vi "LINX - TMP3x.vi"() -> ()   [LabVIEW 2020]
doc: "Read the temperature from a TMP3x sensor."
uses:
  vi.lib/MakerHub/LINX/Public/Utilities/Open Serial.vi
  vi.lib/MakerHub/LINX/Public/Sensors/Temperature/TMP3x/TMP35.vi
  vi.lib/MakerHub/LINX/LMH-LINX.lvlib
  vi.lib/MakerHub/LINX/Private/Device/Device.lvlib
  vi.lib/MakerHub/LINX/Public/Sensors/Temperature/TMP3x/TMP3x.lvlib
panel:
  out "Temp C":dbl(slide) scale=0.0..35.0
  in  "AI Channel":u8
  out "Loop Rate (Hz)":u32
  in  "Stop Button":bool
  in  "Serial Port":refnum<visa-resource-name>
  # "Circuit Schematic"
  # "LINX Device Settings"
  # "Temperature"
  # "Analog Read Example (Serial Interface)\n\nThis example demonstrates how to read analog input values from a LINX device connected to the host computer via Serial / USB.\n\nInstructions\n1. Select the COM Port associated with the LINX Device.\n2. Select the Analog Channel connected to the TMP3x.\n3. Click the Run Arrow."
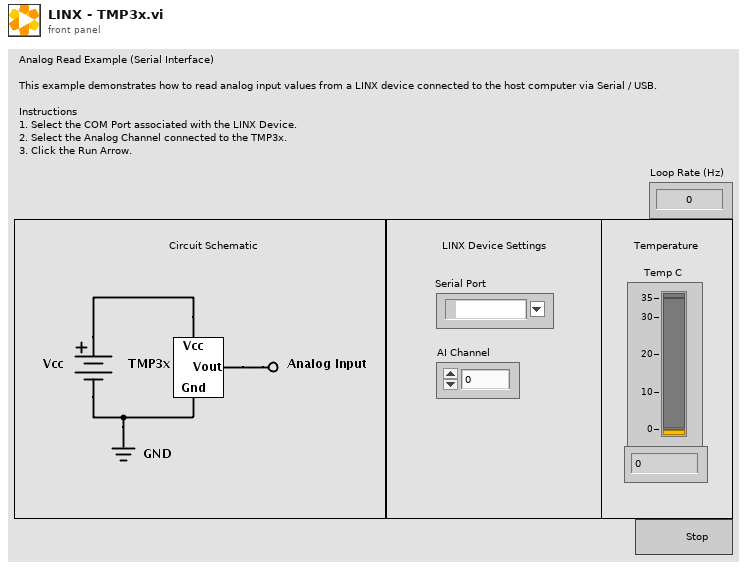
[diagram p1: front panel]
types:
  T1 = typedef "LMH-LINX.lvlib/LINX Ref.ctl" = cluster{"IO":T2, "Interface":T3, "LINX Device Config":T4}
  T2 = typedef "LMH-LINX.lvlib/Platform.ctl" = enum16{"Remote", "Local"}
  T3 = typedef "LMH-LINX.lvlib/Interface.ctl" = enum16{"Serial", "TCP"}
  T4 = typedef "Device.lvlib/LINX Device Config.ctl" = cluster{"Interface":T3, "COM Port":refnum<visa-resource-name>, "TCP Configuration":T5, "Device Family":u8, "Device ID":u8, "Device Name":string, "TCP Ref":refnum<k5>, "Channels":T6}
  T5 = typedef "Device.lvlib/TCP Config.ctl" = cluster{"IP Address":string, "Port":u16}
  T6 = typedef "LMH-LINX.lvlib/Channels.ctl" = cluster{"DI":u8[], "DO":u8[], "AI":u8[], "AO":u8[], "PWM":u8[], "QE":u8[], "UART":u8[], "I2C 2":u8[], "SPI":u8[], "CAN":u8[], "Servo":u8[], "AI Ref (V)":dbl, "AI Resolution (Bits)":u8, "AO Ref (V)":dbl, "AO Resolution (Bits)":u8}
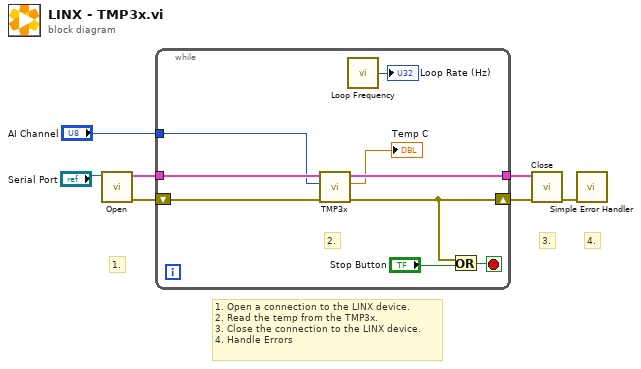
[diagram p0: block diagram]
diagram:
  # "1. Open a connection to the LINX device.\n2. Read the temp from the TMP3x.\n3. Close the connection to the LINX device.\n4. Handle Errors"
  # "4."
  # "3."
  # "1."
  n1 = call-poly "Open.vi"("Serial Port"="Serial Port") -> ("Error Out"=w6:errorcluster, "LINX Resource"=w7:T1)  [unwired: 8 in, 1 out]
  n2 = while {
    tunnel: w7 -> [w12]
    tunnel: [w10] -> w5
    shift-right: [w13] -> w4
    shift-left: w6 -> [w11]
    tunnel: "AI Channel" -> [w9]
    stop <- w16 stop-if-true
    # "2."
    n3 = call-poly "TMP3x.vi"("Error In"=w11, "Analog Channel"=w9, "LINX Resource"=w12) -> ("Error Out"=w13:errorcluster, "Temp C"=→"Temp C":dbl, "LINX Resource"=w10:T1)  [unwired: 6 in]
    n4 = call "Loop Frequency.vi"() -> ("Loop Rate (Hz)"=→"Loop Rate (Hz)":u32)
    n5 = Or(x=w13, y="Stop Button") -> (x .or. y?=w16:bool)
  }
  n6 = call "Close.vi"("Error In"=w4, "LINX Resource"=w5) -> ("Error Out"=w2:errorcluster)  [unwired: 9 in]
  n7 = call <vilib>:"Simple Error Handler.vi"("error in (no error)"=w2) -> ()  [unwired: 4 in, 5 out]
